vi "save stim points.vi"(9 "Stim ref":refnum<vi>, 10 "File Name":string, 11 "path":path) -> (3 "new file path (Not A Path if cancelled)":path)   [LabVIEW 2012]
uses:
  <vilib>/Utility/file.llb/Write To Spreadsheet File (string).vi
panel:
  out "T button?":bool
  # "D:\\gitrepositories\\SciScan\\Parallel Uncaging Module\\Uncaging UI\\Uncaging Dual.vi"
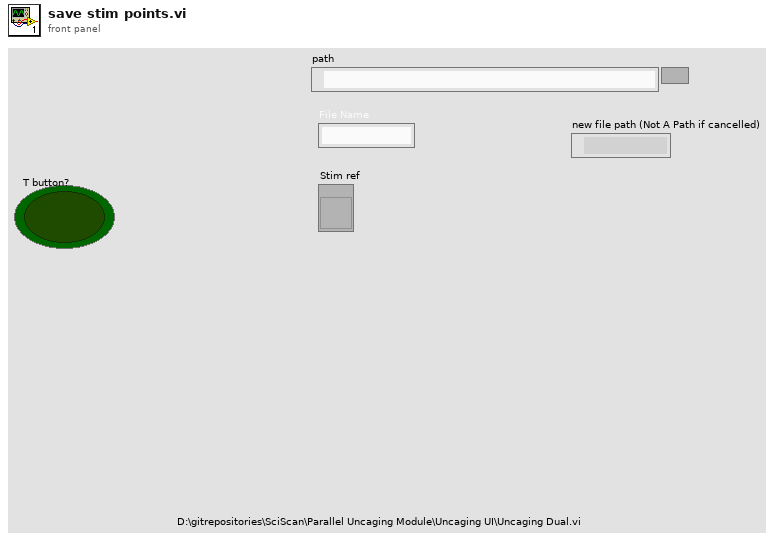
[diagram p1: front panel]
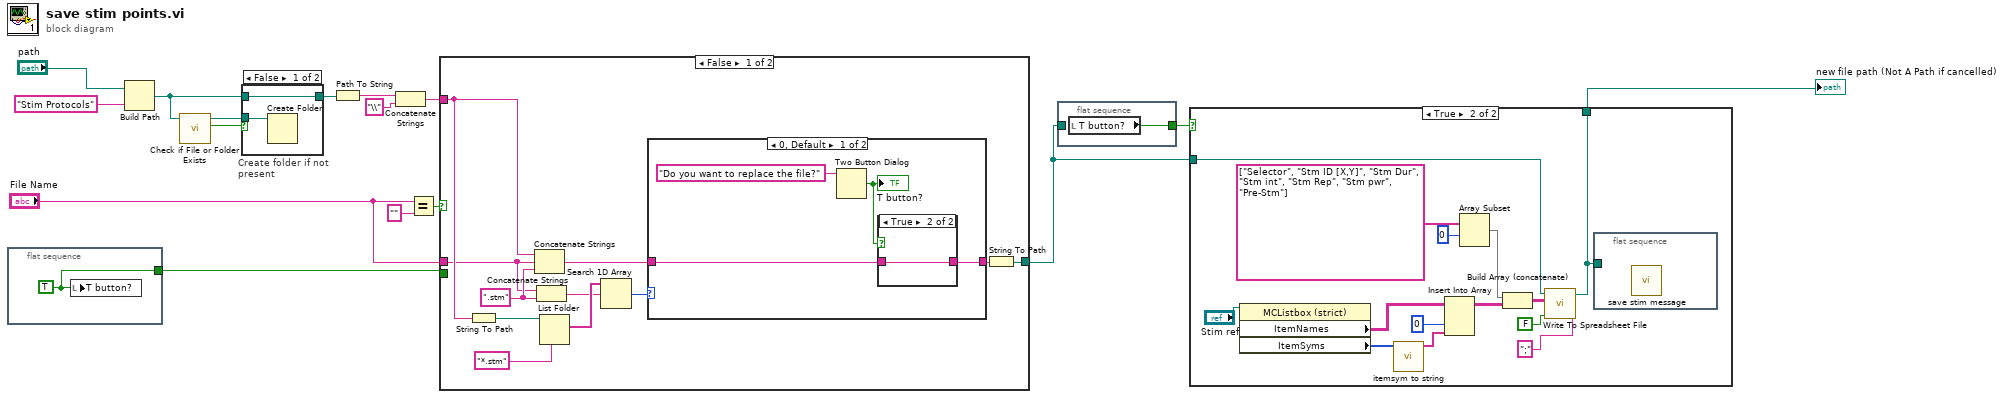
[diagram p0: block diagram]
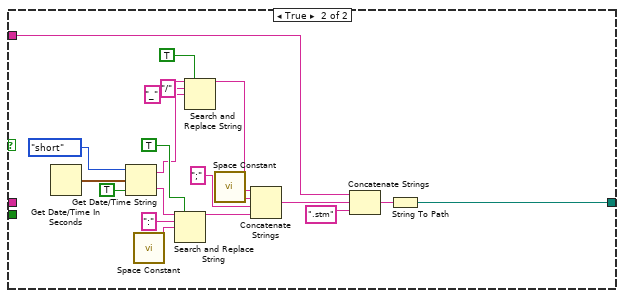
[diagram p6: hidden frame]
diagram:
  n1 = flat-sequence {
    tunnel: [w17] -> w9
    frame #0 {
      w17 = TRUE ("T button?")
      n2 = local write "T button?"(w17) -> ()
    }
  }
  n3 = Build Path(base path="path", name or relative path="Stim Protocols") -> (appended path=w2:path)
  n4 = call <vilib>:"Check if File or Folder Exists.vi"("path"=w2) -> ("file or folder exists?"=w6:bool, "dup path"=w5:path)  [unwired: 8 in, 1 out]
  n5 = case "Create folder if not present" shown="False" w6 {
    tunnel: w2 -> [w18 w20]
    tunnel: [w18 w20] -> w3
    tunnel: w5 -> [w19 _]
    frame False {
      n6 = Create Folder(path (use dialog)=w19) -> ()  [unwired: 2 in, 3 out]
    }
    frame True {
    }
  }
  n7 = Path To String(path=w3) -> (string=w14:string)
  n8 = Concatenate Strings(w14, "\\") -> (w11:string)
  n9 = Equal?(x="File Name", y="" ("File Name")) -> (x = y?=w12:bool)
  n10 = case shown="False" w12 {
    tunnel: "File Name" -> [w21 _]
    tunnel: w11 -> [w22 w46]
    tunnel: [w26 w43] -> w4
    tunnel: w9 -> [_ _]
    frame False {
      w25 = ".stm" ("string")
      n11 = String To Path(string=w22) -> (path=w31:path)
      n12 = Concatenate Strings(w22, w21, w25) -> (w28:string)
      n13 = Concatenate Strings(w21, w25) -> (w24:string)
      n14 = List Folder(path=w31, pattern="*.stm" ("pattern (all files)")) -> (filenames=w30:string[])  [unwired: 2 in, 3 out]
      n15 = Search 1D Array(1D array=w30, element=w24) -> (index of element=w29:i32)  [unwired: 1 in]
      n16 = case shown="0, Default" w29 {
        tunnel: w28 -> [w34 w37]
        tunnel: [w33 w37] -> w27
        frame 0, Default {
          n17 = Two Button Dialog(message="Do you want to replace the file?") -> (T button?=w32:bool)  [unwired: 2 in]
          "T button?" <- w32
          n18 = case shown="True" w32 {
            tunnel: w34 -> [_ w36]
            tunnel: [_ w36] -> w33
            frame False {
            }
            frame True {
            }
          }
        }
        frame -1 {
        }
      }
      n19 = String To Path(string=w27) -> (path=w26:path)
    }
    frame True {
      n20 = Get Date/Time In Seconds() -> (seconds since 1Jan1904=w56:timestamp)
      n21 = Get Date/Time String(date format (0)=enum16{"short", "long", "abbreviated"}."short", seconds (now)=w56, want seconds? (F)=TRUE) -> (date string=w42:string, time string=w50:string)
      n22 = call <vilib>:"Space Constant.vi"() -> ("String"=w51:string)
      n23 = Search and Replace String(replace all?=TRUE ("replace all? (F)"), input string=w50, search string=":", replace string=w51) -> (result string=w49:string)  [unwired: 4 in, 3 out]
      n24 = Search and Replace String(replace all?=TRUE ("replace all? (F)"), input string=w42, search string="/", replace string="_" ("replace string (\"\")")) -> (result string=w39:string)  [unwired: 4 in, 3 out]
      n25 = call <vilib>:"Space Constant.vi"() -> ("String"=w48:string)
      n26 = Concatenate Strings(w48, w39, ";" ("string"), w49) -> (w45:string)
      n27 = Concatenate Strings(w46, w45, ".stm" ("string")) -> (w57:string)
      n28 = String To Path(string=w57) -> (path=w43:path)
    }
  }
  n29 = flat-sequence {
    tunnel: [w58] -> w8
    tunnel: w4 -> [_]
    frame #0 {
      n30 = local read "T button?"() -> (w58:bool)
    }
  }
  n31 = case shown="True" w8 {
    tunnel: w4 -> [_ w71]
    tunnel: [_ w59] -> w7
    frame False {
    }
    frame True {
      n32 = property on="Property Node" class="MCListbox (strict)"(reference="Stim ref") -> ("ItemNames"=w65:string[][], "ItemSyms"=w67:i32[])  [unwired: 1 in, 2 out]
      n33 = call "itemsym to string.vi"("Item sym"=w67) -> ("Item sym string"=w64:string[])  [unwired: 10 in]
      n34 = Insert Into Array(array=w65, index (col)=0 ("disabled index (col)"), new element=w64) -> (w62:string[][])  [unwired: 1 in]
      n35 = Array Subset(array=string[] ["Selector", "Stm ID [X,Y]", "Stm Dur", "Stm int", "Stm Rep", "Stm pwr", "Pre-Stm"] ("ColHdrString"), index=0) -> (w66:string[])  [unwired: 1 in]
      n36 = Build Array (concatenate)(w66, w62) -> (w61:string[][])
      n37 = call-poly <vilib>:"Write To Spreadsheet File.vi"("delimiter (\\t)"=";" ("delimiter (\\t)"), "append to file? (new file:F)"=FALSE, "2D data"=w61, "file path (dialog if empty)"=w71) -> ("new file path (Not A Path if cancelled)"=w59:path)  [unwired: 4 in]
      n38 = flat-sequence {
        tunnel: w59 -> [_]
        frame #0 {
          n39 = call "save stim message.vi"() -> ()  [unwired: 12 in]
        }
      }
    }
  }
  "new file path (Not A Path if cancelled)" <- w7
